vi "MAVLink Attitude.vi"(7 "FGV Method":T2, 11 "Attitude":T1) -> (3 "Attitude out":T1)   [LabVIEW 2014]
uses:
  Controls/FGV Methods.ctl
  MAVLink/Controls/MAVLink Attitude.ctl
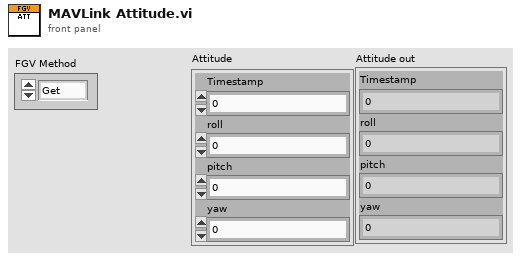
[diagram p1: front panel]
types:
  T1 = typedef "MAVLink Attitude.ctl" = cluster{"Timestamp":u32, "roll":sgl, "pitch":sgl, "yaw":sgl}
  T2 = typedef "FGV Methods.ctl" = enum16{"Get", "Set"}
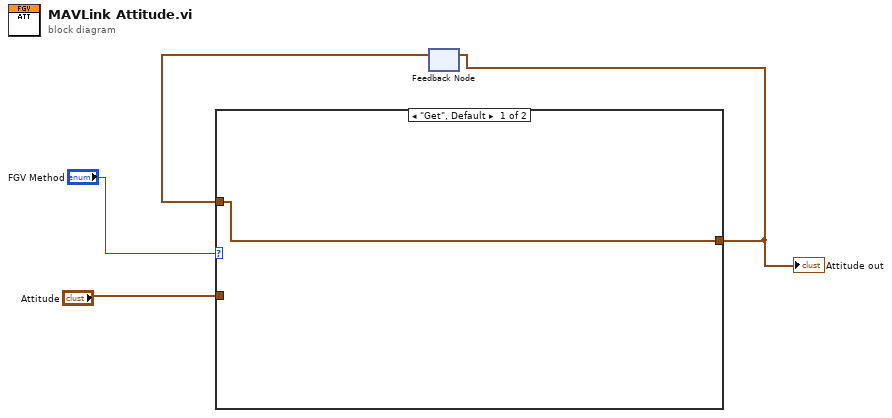
[diagram p0: block diagram]
diagram:
  n1 = feedback #1() -> (w2:T1)  [unwired: 1 in]
  n2 = case shown="\"Get\", Default" "FGV Method" {
    tunnel: "Attitude" -> [_ w6]
    tunnel: [w5 w6] -> w3
    tunnel: w2 -> [w5 _]
    frame "Get", Default {
    }
    frame "Set" {
    }
  }
  "Attitude out" <- w3
  n3 = feedback-in #1(w3) -> ()
